vi "Waveform Page.vi"(8 "error in":errorcluster, 11 "Node Ptr":T1 format="%.0x") -> (0 "error out":errorcluster)   [LabVIEW 2026]
uses:
  <vilib>/NI VeriStand/Custom Device API/Custom Device Item Ref.ctl
  C:/Program Files/National Instruments/VeriStand 2026/NationalInstruments.VeriStand.Controls.dll
  Program Files/National Instruments/VeriStand 2026/NationalInstruments.VeriStand.Controls.dll
  <vilib>/NI VeriStand/Custom Device API/Custom Device API.lvlib
panel:
  in  "PagePropertyEditor":refnum<k24>(container)
  out "Waveform":string[][](table) caption="Waveform Settings"
  in  "General Header":cluster{"Section Name":string}={"Section Name"="Waveform Settings"}
  in  "Description":string
  in  "Name":string
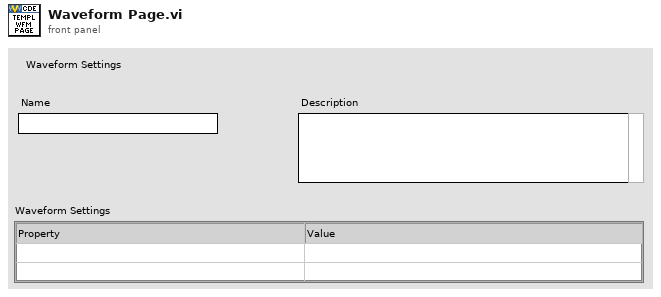
[diagram p1: front panel]
types:
  T1 = typedef "Custom Device API.lvlib/Custom Device Item Ref.ctl" = u64
  T2 = typedef "Custom Device API.lvlib/Custom Device Item Info.ctl" = cluster{"Name":string, "Is Channel":bool, "GUID":string, "Is Waveform":bool}
  T3 = typedef "Custom Device API.lvlib/Custom Device Commands.ctl" = enum16{"Default", "Item renamed", "Shutdown", "Dynamic button pressed"}
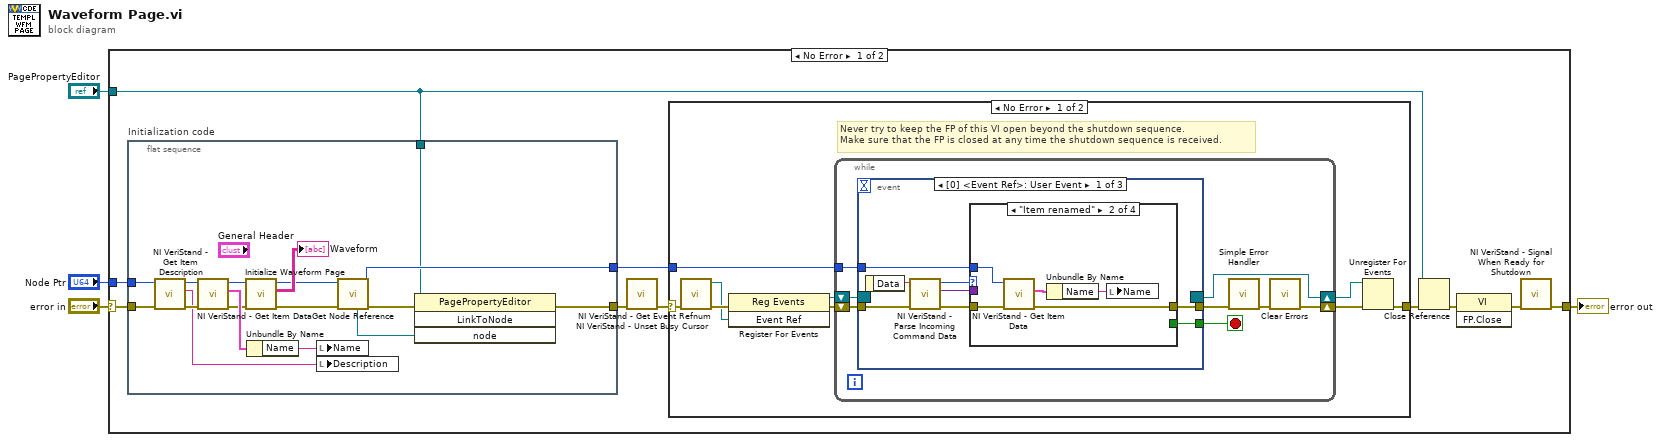
[diagram p0: block diagram]
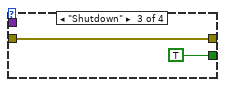
[diagram p3: hidden frame]
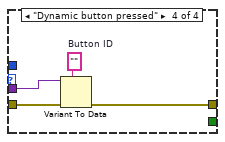
[diagram p4: hidden frame]
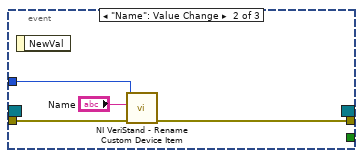
[diagram p5: hidden frame]
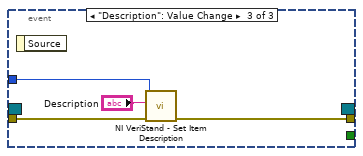
[diagram p6: hidden frame]
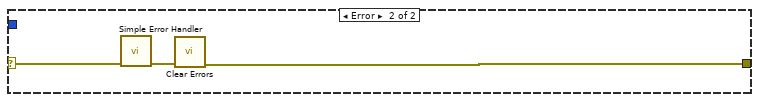
[diagram p7: hidden frame]
diagram:
  n1 = case shown="No Error" "error in" {
    selector: "error in" -> [w9 w80]
    tunnel: [w14 w80] -> w2
    tunnel: "Node Ptr" -> [w8 _]
    tunnel: "PagePropertyEditor" -> [w7 _]
    frame No Error {
      n2 = flat-sequence "Initialization code" {
        tunnel: w9 -> [w30]
        tunnel: w8 -> [w27]
        tunnel: [w19] -> w10
        tunnel: [w18] -> w11
        tunnel: w7 -> [w16]
        frame #0 {
          n3 = call <vilib>:"NI VeriStand - Get Item Description.vi"("error in (no error)"=w30, "Item Ref in"=w27) -> ("error out"=w31:errorcluster, "Description"=w25:string, "Item Ref out"=w29:T1)  [unwired: 7 out]
          n4 = call <vilib>:"NI VeriStand - Get Item Data.vi"("error in (no error)"=w31, "Item Ref in"=w29) -> ("error out"=w24:errorcluster, "Item Info"=w28:T2, "Item Ref out"=w23:T1)  [unwired: 7 out]
          n5 = call "Initialize Waveform Page.vi"("error in"=w24, "Node Ptr"=w23) -> ("error out"=w20:errorcluster, "Waveform Settings Table"=→"Waveform":string[][], "Node Ptr out"=w17:T1)  [unwired: 7 in]
          n6 = Unbundle By Name(w28) -> ("Name"=w26:string)
          n7 = local write "Name"(w26) -> ()
          n8 = local write "Description"(w25) -> ()
          n9 = call "Get Node Reference.vi"("error in"=w20, "Node Ptr"=w17) -> ("error out"=w21:errorcluster, "Node Ptr"=w18:T1, "Base Node"=w15:refnum<k24>)  [unwired: 6 in, 1 out]
          n10 = invoke class="PagePropertyEditor" method="LinkToNode"(reference=w16, error in=w21, "node"=w15) -> (error out=w19:errorcluster)  [unwired: 1 in, 3 out]
        }
      }
      n11 = call <vilib>:"NI VeriStand - Unset Busy Cursor.vi"("error in (no error)"=w10) -> ("error out"=w12:errorcluster)  [unwired: 10 out]
      n12 = case shown="No Error" w12 {
        selector: w12 -> [w36 w79]
        tunnel: [w38 w77] -> w6
        tunnel: w11 -> [w32 _]
        frame No Error {
          # "Never try to keep the FP of this VI open beyond the shutdown sequence.\nMake sure that the FP is closed at any time the shutdown sequence is received."
          n13 = call <vilib>:"NI VeriStand - Get Event Refnum.vi"("error in (no error)"=w36) -> ("error out"=w40:errorcluster, "Event Ref"=w34:refnum<user-event>)  [unwired: 9 out]
          n14 = register-events(error in=w40, w34) -> (reference out=w33:refnum<event-registration>, error out=w37:errorcluster)  [unwired: 1 in]
          n15 = while {
            tunnel: w32 -> [w41]
            shift-right: [w45] -> w39
            shift-left: w37 -> [w48]
            shift-right: [w44] -> w35
            shift-left: w33 -> [w43]
            stop <- w42 stop-if-true
            n16 = event shown="[0] <Event Ref>: User Event" {
              selector: w43 -> [_ _ _]
              dyn-events: [_ _ _] -> w44
              timeout: _ -> [_ _ _]
              tunnel: w48 -> [w56 w72 w76]
              tunnel: [w51 _ _] -> w42
              tunnel: [w54 w71 w75] -> w47
              tunnel: w41 -> [w50 w70 w74]
              event User Event {
                n17 = event-data() -> ("Data"=w53:string)  [unwired: 1 out]
                n18 = call <vilib>:"NI VeriStand - Parse Incoming Command Data.vi"("error in (no error)"=w56, "Incoming data"=w53) -> ("error out"=w55:errorcluster, "Outgoing data"=w49:variant, "Action"=w52:T3)  [unwired: 7 out]
                n19 = case shown="\"Item renamed\"" w52 {
                  tunnel: w55 -> [w57 w62 w64 w68]
                  tunnel: [_ _ TRUE _] -> w51
                  tunnel: [w57 w61 w64 w67] -> w54
                  tunnel: w50 -> [_ w60 _ _]
                  tunnel: w49 -> [_ _ _ w66]
                  frame "Default", Default {
                  }
                  frame "Item renamed" {
                    n20 = call <vilib>:"NI VeriStand - Get Item Data.vi"("error in (no error)"=w62, "Item Ref in"=w60) -> ("error out"=w61:errorcluster, "Item Info"=w59:T2)  [unwired: 8 out]
                    n21 = Unbundle By Name(w59) -> ("Name"=w58:string)
                    n22 = local write "Name"(w58) -> ()
                  }
                  frame "Shutdown" {
                  }
                  frame "Dynamic button pressed" {
                    w65 = ""  # Button ID
                    n23 = Variant To Data(error in=w68, type=w65, Variant=w66) -> (error out=w67:errorcluster)  [unwired: 1 out]
                  }
                }
              }
              event "Name": Value Change {
                n24 = event-data() -> ()  [unwired: 2 out]
                n25 = call <vilib>:"NI VeriStand - Rename Custom Device Item.vi"("error in (no error)"=w72, "New Name"="Name", "Item Ref in"=w70) -> ("error out"=w71:errorcluster)  [unwired: 1 in, 7 out]
              }
              event "Description": Value Change {
                n26 = event-data() -> ()  [unwired: 2 out]
                n27 = call <vilib>:"NI VeriStand - Set Item Description.vi"("error in (no error)"=w76, "Description"="Description", "Item Ref in"=w74) -> ("error out"=w75:errorcluster)  [unwired: 8 out]
              }
            }
            n28 = call <vilib>:"Simple Error Handler.vi"("error in (no error)"=w47) -> ("error out"=w46:errorcluster)  [unwired: 1 in, 7 out]
            n29 = call <vilib>:"Clear Errors.vi"("error in (no error)"=w46) -> ("error out"=w45:errorcluster)  [unwired: 1 in, 5 out]
          }
          n30 = Unregister For Events(event registration refnum=w35, error in=w39) -> (error out=w38:errorcluster)
        }
        frame Error {
          n31 = call <vilib>:"Simple Error Handler.vi"("error in (no error)"=w79) -> ("error out"=w78:errorcluster)  [unwired: 1 in, 7 out]
          n32 = call <vilib>:"Clear Errors.vi"("error in (no error)"=w78) -> ("error out"=w77:errorcluster)  [unwired: 1 in, 5 out]
        }
      }
      n33 = Close Reference(reference=w7, error in (no error)=w6) -> (error out=w5:errorcluster)
      n34 = invoke class="VI" method="FP.Close"(error in=w5) -> (error out=w13:errorcluster)  [unwired: 2 in, 2 out]
      n35 = call <vilib>:"NI VeriStand - Signal When Ready for Shutdown.vi"("error in (no error)"=w13) -> ("error out"=w14:errorcluster)  [unwired: 10 out]
    }
    frame Error {
    }
  }
  "error out" <- w2
